vi "Database_User_Read.vi"(8 "error in":errorcluster, 9 "Language":T2, 10 "ID_Number":string, 11 "connection reference":T1) -> (0 "error out":errorcluster, 1 "Ok?":bool, 2 "Message":string, 3 "UserRight":T3)   [LabVIEW 2015]
uses:
  CustomControl/UserRight.ctl
  CustomControl/Lang_Control.ctl
  <vilib>/addons/database/Connection.llb/Conn ObjectReference.ctl
  <vilib>/addons/database/Connection.llb/Conn Execute.vi
  <vilib>/addons/database/Recordset.llb/Rec Fetch Recordset Data (R).vi
  <vilib>/addons/database/Recordset.llb/Rec Destroy - Connection.vi
  <vilib>/addons/database/_DB Variant To Data/Database Variant To Data.xnode
  <vilib>/addons/database/NI_Database_API.lvlib
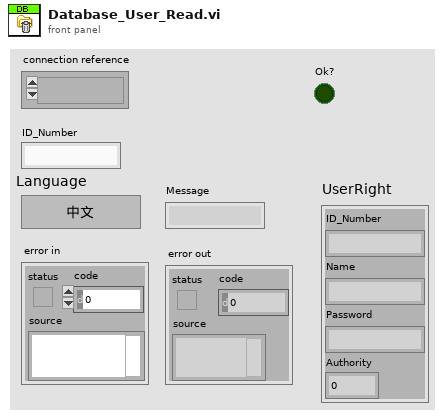
[diagram p1: front panel]
types:
  T1 = typedef "NI_Database_API.lvlib/Conn ObjectReference.ctl" = refnum<k1>
  T2 = typedef "Lang_Control.ctl" = enum16{"中文", "English"}
  T3 = typedef "UserRight.ctl" = cluster{"ID_Number":string, "Name":string, "Password":string, "Authority":i32}
  T4 = typedef "NI_Database_API.lvlib/Rec ObjectReference.ctl" = refnum<k1>
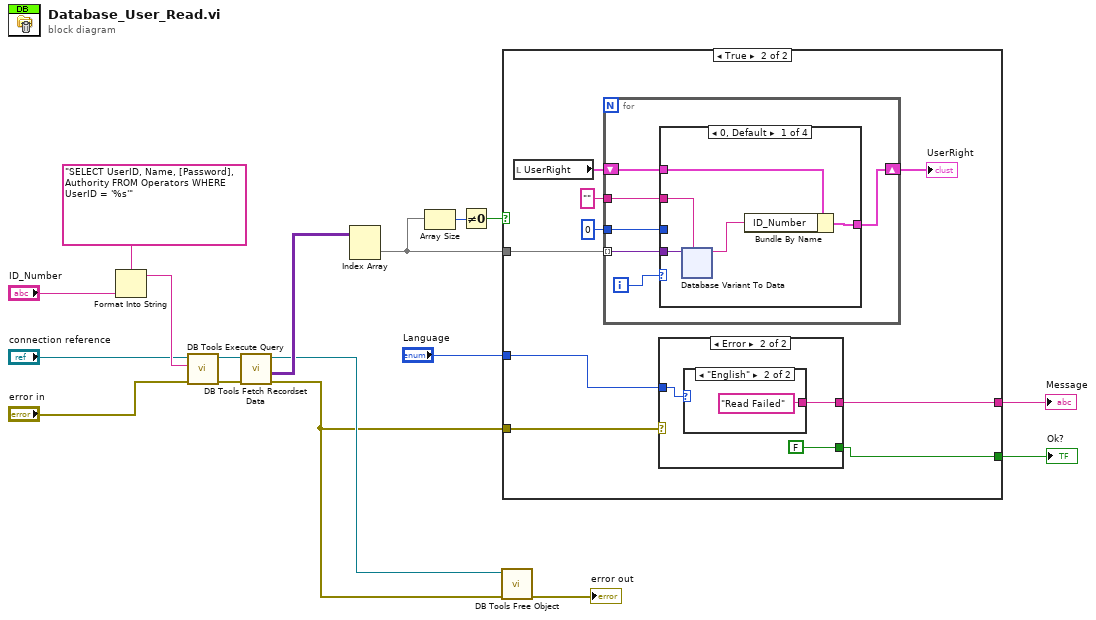
[diagram p0: block diagram]
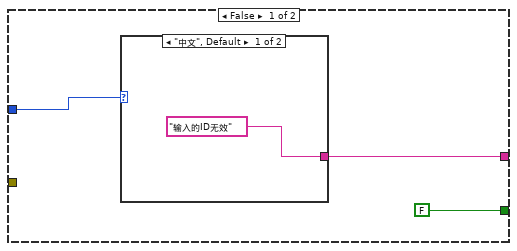
[diagram p2: hidden frame]
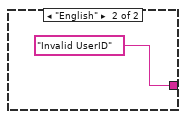
[diagram p3: hidden frame]
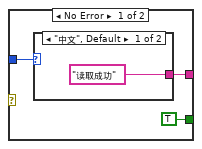
[diagram p4: hidden frame]
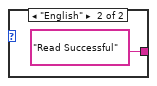
[diagram p5: hidden frame]
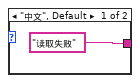
[diagram p6: hidden frame]
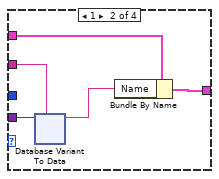
[diagram p7: hidden frame]
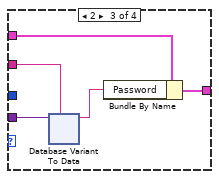
[diagram p8: hidden frame]
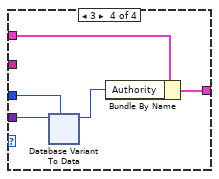
[diagram p9: hidden frame]
diagram:
  n1 = Format Into String(format string="SELECT UserID, Name, [Password], Authority FROM Operators WHERE UserID = '%s'", "ID_Number") -> (resulting string=w15:string)  [unwired: 2 in, 1 out]
  n2 = call-poly <vilib>:"DB Tools Execute Query.vi"("error in (no error)"="error in", "SQL query"=w15, "connection reference"="connection reference") -> ("error out"=w14:errorcluster, "recordset reference"=w13:T4)  [unwired: 5 in]
  n3 = call-poly <vilib>:"DB Tools Fetch Recordset Data.vi"("error in (no error)"=w14, "recordset reference"=w13) -> ("error out"=w4:errorcluster, "recordset data"=w12:variant[][], "recordset reference out"=w9:T4)  [unwired: 3 in]
  n4 = Index Array(array=w12) -> (element=w8:variant[])  [unwired: 2 in]
  n5 = Array Size(array=w8) -> (size(s)=w6:i32)
  n6 = Not Equal To 0?(x=w6) -> (x != 0?=w7:bool)
  n7 = call-poly <vilib>:"DB Tools Free Object.vi"("error in (no error)"=w4, "recordset reference"=w9) -> ("error out"=→"error out":errorcluster)  [unwired: 8 in, 1 out]
  n8 = case shown="True" w7 {
    tunnel: w8 -> [_ w30]
    tunnel: w4 -> [_ w26]
    tunnel: [w19 w25] -> w2
    tunnel: "Language" -> [w20 w24]
    tunnel: [FALSE ("Ok?") w23] -> w1
    frame False {
      n9 = case shown="\"中文\", Default" w20 {
        tunnel: ["输入的ID无效" "Invalid UserID"] -> w19
        frame "中文", Default {
        }
        frame "English" {
        }
      }
    }
    frame True {
      n10 = local read "UserRight"() -> (w27:T3)
      n11 = for {
        tunnel: w30 -> [w46] mode=indexing
        tunnel: 0 -> [w45]
        tunnel: "" ("userID") -> [w44]
        shift-right: [w42] -> w31
        shift-left: w27 -> [w43]
        i -> [w47]
        n12 = case shown="0, Default" w47 {
          tunnel: w46 -> [w52 w89 w126 w163]
          tunnel: w45 -> [_ _ _ w160]
          tunnel: w44 -> [w48 w88 w125 _]
          tunnel: w43 -> [w51 w86 w123 w161]
          tunnel: [w49 w87 w124 w162] -> w42
          frame 0, Default {
            n13 = xnode "Database Variant To Data"("database variant"=w52, "type"=w48) -> ("data"=w50:string)  [unwired: 1 in, 1 out]
            n14 = Bundle By Name(cluster=w51, "ID_Number"=w50) -> (w49:T3)
          }
          frame 1 {
            n15 = xnode "Database Variant To Data"("database variant"=w89, "type"=w88) -> ("data"=w85:string)  [unwired: 1 in, 1 out]
            n16 = Bundle By Name(cluster=w86, "Name"=w85) -> (w87:T3)
          }
          frame 2 {
            n17 = xnode "Database Variant To Data"("database variant"=w126, "type"=w125) -> ("data"=w122:string)  [unwired: 1 in, 1 out]
            n18 = Bundle By Name(cluster=w123, "Password"=w122) -> (w124:T3)
          }
          frame 3 {
            n19 = xnode "Database Variant To Data"("database variant"=w163, "type"=w160) -> ("data"=w159:i32)  [unwired: 1 in, 1 out]
            n20 = Bundle By Name(cluster=w161, "Authority"=w159) -> (w162:T3)
          }
        }
      }
      "UserRight" <- w31
      n21 = case shown="Error" w26 {
        tunnel: w24 -> [w34 w39]
        tunnel: [w33 w38] -> w25
        tunnel: [TRUE ("Ok?") FALSE ("Ok?")] -> w23
        frame No Error {
          n22 = case shown="\"中文\", Default" w34 {
            tunnel: ["读取成功" "Read Successful"] -> w33
            frame "中文", Default {
            }
            frame "English" {
            }
          }
        }
        frame Error {
          n23 = case shown="\"English\"" w39 {
            tunnel: ["读取失败" "Read Failed"] -> w38
            frame "中文", Default {
            }
            frame "English" {
            }
          }
        }
      }
    }
  }
  "Message" <- w2
  "Ok?" <- w1
